vi "Get All Process Names.vi"(8 "错误输入（无错误）":errorcluster) -> (0 "错误输出":errorcluster, 3 "ProcessNames":string[](array[string]))   [LabVIEW 2011]
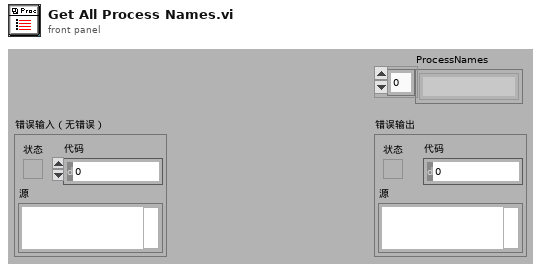
[diagram p1: front panel]
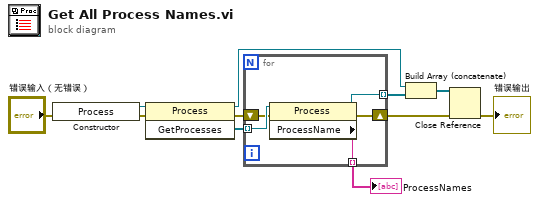
[diagram p0: block diagram]
diagram:
  n1 = constructor class="Process"(error in="错误输入（无错误）") -> (reference out=w11:refnum<k24>, error out=w10:errorcluster)  [unwired: 2 in, 1 out]
  n2 = invoke class="Process" method="GetProcesses"(reference=w11, error in=w10) -> (reference out=w6:refnum<k24>, error out=w7:errorcluster, "GetProcesses"=w9:refnum<k24>[])  [unwired: 1 in]
  n3 = for {
    tunnel: w9 -> [w16] mode=indexing
    tunnel: [w15] -> w5 mode=indexing
    tunnel: [w14] -> w8 mode=indexing
    shift-right: [w12] -> w4
    shift-left: w7 -> [w13]
    n4 = property class="Process"(reference=w16, error in=w13) -> (reference out=w15:refnum<k24>, error out=w12:errorcluster, "ProcessName"=w14:string)
  }
  "ProcessNames" <- w8
  n5 = Build Array (concatenate)(w6, w5) -> (w3:refnum<k24>[])
  n6 = Close Reference(reference=w3, error in (no error)=w4) -> (error out=→"错误输出":errorcluster)
